vi "Module New.vi"(7 "Parent ID":i32, 8 "error in (no error)":errorcluster, 9 "Config Section":string, 10 "Config Path":path, 11 "Name":string) -> (0 "error out":errorcluster, 3 "Module":T1)   [LabVIEW 2022 SP3, in "Core.lvlib"]
uses:
  Core.lvlib
  Controls/Module Instance.ctl
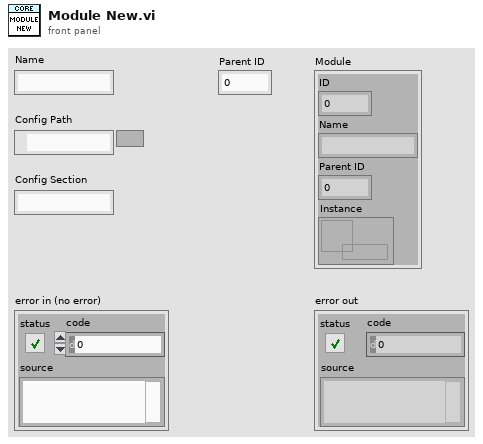
[diagram p1: front panel]
types:
  T1 = cluster{"ID":i32, "Name":string, "Parent ID":i32, "Instance":refnum<data-value>}
  T2 = typedef "Core.lvlib/Module Instance.ctl" = cluster{"Queue":refnum<queue>, "Config Path":path, "Config Section":string}
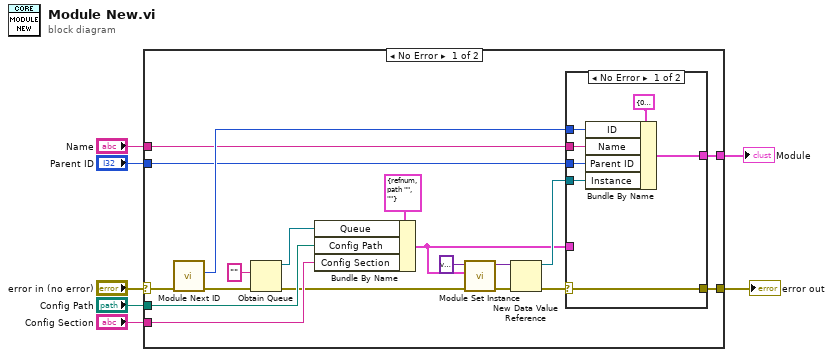
[diagram p0: block diagram]
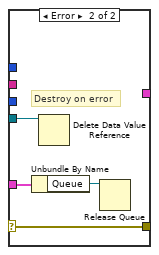
[diagram p2: hidden frame]
diagram:
  n1 = case shown="No Error" "error in (no error)" {
    selector: "error in (no error)" -> [w26 w38]
    tunnel: [w25 w38] -> w6
    tunnel: "Parent ID" -> [w21 _]
    tunnel: "Name" -> [w22 _]
    tunnel: "Config Path" -> [w16 _]
    tunnel: "Config Section" -> [w15 _]
    tunnel: [w24 _] -> w1
    frame No Error {
      n2 = call "Module Next ID.vi"("error in (no error)"=w26) -> ("error out"=w17:errorcluster, "Next ID"=w23:i32)  [unwired: 8 in, 1 out]
      n3 = Obtain Queue(element data type="", error in (no error)=w17) -> (queue out=w20:refnum<queue>, error out=w12:errorcluster)  [unwired: 3 in, 1 out]
      n4 = Bundle By Name(cluster=T2 {"Queue"=refnum, "Config Path"=path "", "Config Section"=""} ("Module Data"), "Queue"=w20, "Config Path"=w16, "Config Section"=w15) -> (w8:T2)
      n5 = call "Module Set Instance.vi"("error in (no error)"=w12, "Instance"=w8, "Self in"=variant ("Self")) -> ("error out"=w11:errorcluster, "Self out"=w13:variant)  [unwired: 7 in]
      n6 = New Data Value Reference(data value=w13, error in=w11) -> (data value reference=w9:refnum<data-value>, error out=w10:errorcluster)
      n7 = case shown="No Error" w10 {
        selector: w10 -> [w33 w37]
        tunnel: [w33 w37] -> w25
        tunnel: [w29 _] -> w24
        tunnel: w23 -> [w32 _]
        tunnel: w22 -> [w31 _]
        tunnel: w21 -> [w30 _]
        tunnel: w9 -> [w27 w36]
        tunnel: w8 -> [_ w35]
        frame No Error {
          n8 = Bundle By Name(cluster=T1 {"ID"=0, "Name"="", "Parent ID"=0, "Instance"=refnum} ("Module"), "ID"=w32, "Name"=w31, "Parent ID"=w30, "Instance"=w27) -> (w29:T1)
        }
        frame Error {
          # "Destroy on error"
          n9 = Unbundle By Name(w35) -> ("Queue"=w34:refnum<queue>)
          n10 = Delete Data Value Reference(data value reference=w36) -> ()  [unwired: 1 in, 2 out]
          n11 = Release Queue(queue=w34) -> ()  [unwired: 2 in, 3 out]
        }
      }
    }
    frame Error {
    }
  }
  "error out" <- w6
  "Module" <- w1
